vi "VLC-IP_Enqueue_Images.vi"(0 "VLC-IP":T1, 1 "dTime":refnum<vi>, 5 "Stop in":refnum<vi>, 7 "queue in":refnum<queue>, 11 "error in (no error)":errorcluster) -> (15 "error out":errorcluster)   [LabVIEW 2016]
uses:
  <vilib>/vision/Image Controls.llb/IMAQ Image.ctl
  VLC-IP.ctl
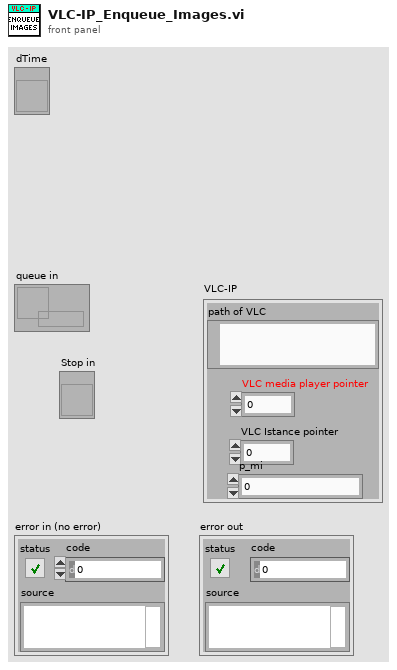
[diagram p1: front panel]
types:
  T1 = typedef "VLC-IP.ctl" = cluster{"path of VLC":path, "VLC media player pointer":i32, "VLC Istance pointer":i32, "p_mi":i32}
  T2 = typedef "Image Type" = u32
  T3 = typedef "IMAQ Image.ctl" = refnum<image>
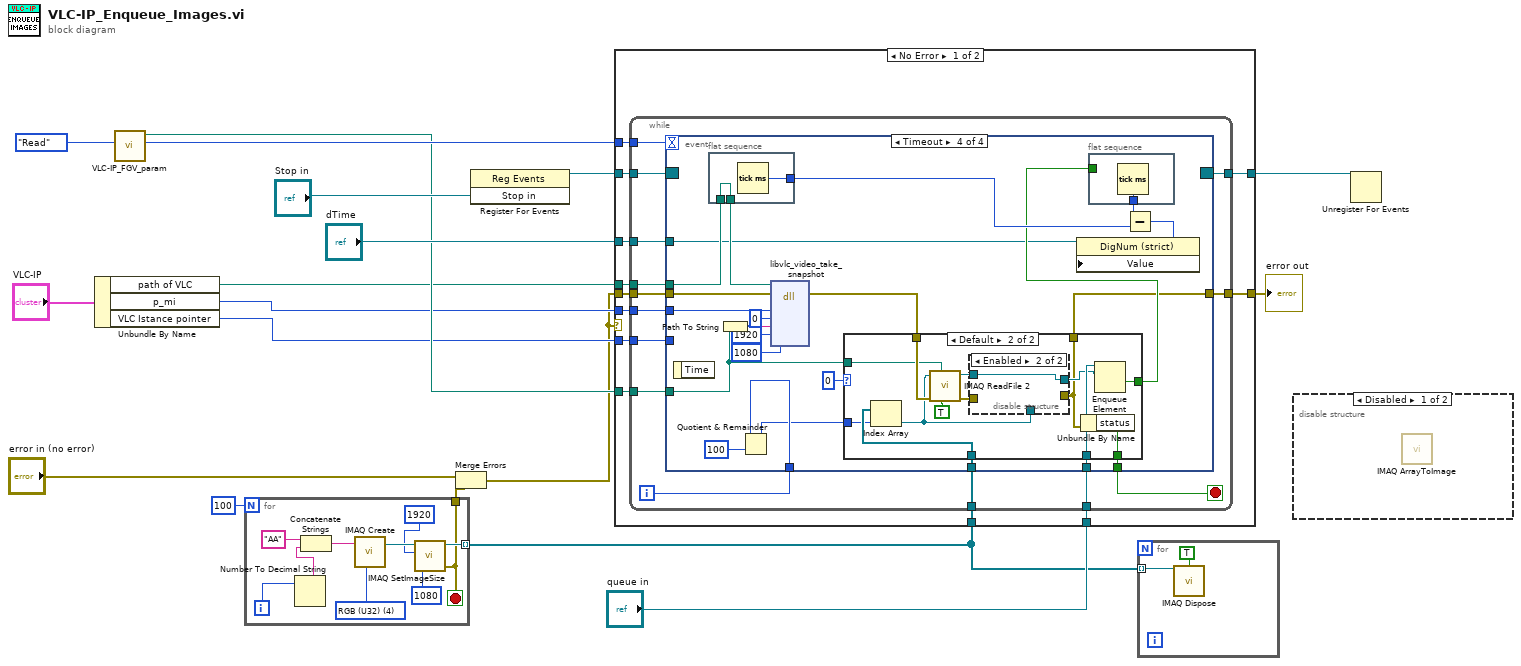
[diagram p0: block diagram]
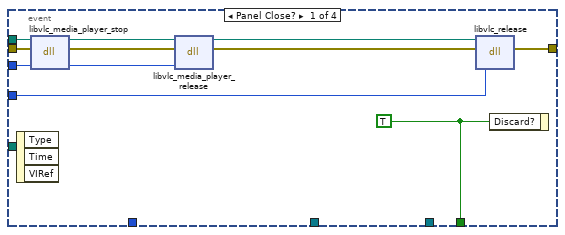
[diagram p3: hidden frame]
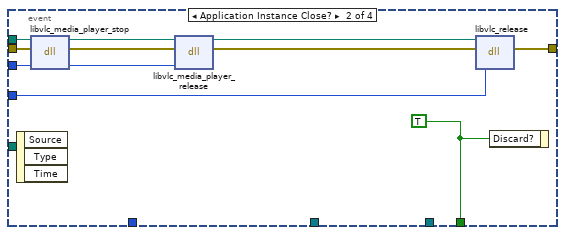
[diagram p4: hidden frame]
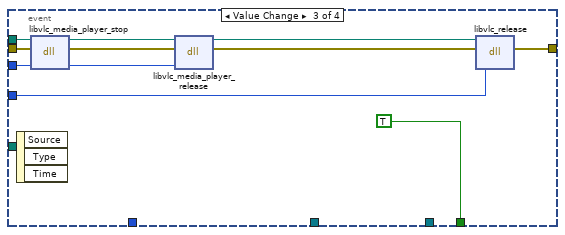
[diagram p5: hidden frame]
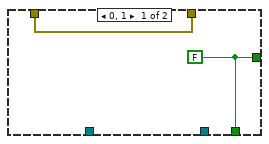
[diagram p6: hidden frame]
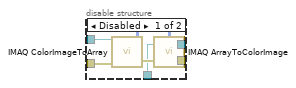
[diagram p7: hidden frame]
diagram:
  n1 = Unbundle By Name("VLC-IP") -> ("path of VLC"=w7:path, "p_mi"=w5:i32, "VLC Istance pointer"=w6:i32)
  n2 = call "VLC-IP_FGV_param.vi"("Mode"=enum16{"Read", "Write"}."Read") -> ("SamplingTime_out"=w10:i32, "TemporaryFilePath_out"=w9:path)  [unwired: 9 in]
  n3 = for {
    N: 100 -> [_]
    tunnel: [w22] -> w3 mode=indexing
    tunnel: [w19] -> w1
    i -> [w24]
    stop <- w19 stop-if-true
    w28 = T2 4 items=["Grayscale (U8)", "Grayscale (I16)", "Grayscale (SGL)", "Complex (CSG)", "RGB (U32)", "HSL (U32)", "RGB (U64)", "Grayscale (U16)"] ("Image Type")
    n4 = Number To Decimal String(number=w24) -> (decimal integer string=w25:string)  [unwired: 1 in]
    n5 = Concatenate Strings("AA" ("Image Name"), w25) -> (w26:string)
    n6 = call "IMAQ Create"("Image Name"=w26, "Image Type"=w28) -> ("New Image"=w21:T3)  [unwired: 3 in, 1 out]
    n7 = call "IMAQ SetImageSize"("Y Resolution"=1080, "X Resolution"=1920, "Image"=w21) -> ("error out"=w19:errorcluster, "Image Out"=w22:T3)  [unwired: 2 in]
  }
  n8 = Merge Errors("error in (no error)", w1) -> (w2:errorcluster)
  n9 = register-events("Stop in") -> (reference out=w15:refnum<event-registration>)  [unwired: 2 in, 1 out]
  n10 = case shown="No Error" w2 {
    tunnel: w6 -> [w40 _]
    tunnel: w5 -> [w39 _]
    tunnel: w2 -> [w38 w138]
    tunnel: w7 -> [w37 _]
    tunnel: [w36 w138] -> w12
    tunnel: w9 -> [w35 _]
    tunnel: w3 -> [w34 _]
    tunnel: "queue in" -> [w33 _]
    tunnel: w10 -> [w32 _]
    tunnel: w15 -> [w31 w137]
    tunnel: [w30 w137] -> w16
    tunnel: "dTime" -> [w29 _]
    frame No Error {
      n11 = while {
        tunnel: w40 -> [w54]
        tunnel: w39 -> [w53]
        tunnel: w38 -> [w52]
        tunnel: w37 -> [w51]
        tunnel: [w50] -> w36
        tunnel: w35 -> [w48]
        tunnel: w34 -> [w47]
        tunnel: w33 -> [w46]
        tunnel: w32 -> [w44]
        tunnel: w31 -> [w43]
        tunnel: [w42] -> w30
        tunnel: w29 -> [w41]
        i -> [w45]
        stop <- w49 stop-if-true
        n12 = event shown="[3] Timeout" {
          selector: w43 -> [_ _ _ _]
          dyn-events: [_ _ _ _] -> w42
          timeout: w44 -> [_ _ _ _]
          tunnel: w52 -> [w65 w76 w87 w106]
          tunnel: w53 -> [w64 w75 w86 w105]
          tunnel: w54 -> [w60 w71 w82 _]
          tunnel: w51 -> [w59 w70 w81 w98]
          tunnel: [w56 w67 w78 w89] -> w50
          tunnel: [w55 w66 TRUE ("Discard?") w90] -> w49
          tunnel: w48 -> [_ _ _ w99]
          tunnel: w47 -> [_ _ _ w101]
          tunnel: w46 -> [_ _ _ w100]
          tunnel: w45 -> [_ _ _ w93]
          tunnel: w41 -> [_ _ _ w95]
          event Panel Close? {
            w55 = TRUE ("Discard?")
            n13 = event-data() -> ()  [unwired: 1 in, 3 out]
            n14 = dll-call lib="C:/Program Files (x86)/VideoLAN/VLC/libvlc.dll" fn="libvlc_media_player_stop"(path in=w59, error in=w65, "p_mi"=w64) -> (path out=w58:path, error out=w63:errorcluster, "p_mi"=w62:i32)  [unwired: 2 in]
            n15 = dll-call lib="C:/Program Files (x86)/VideoLAN/VLC/libvlc.dll" fn="libvlc_media_player_release"(path in=w58, error in=w63, "p_mi"=w62) -> (path out=w57:path, error out=w61:errorcluster)  [unwired: 3 in]
            n16 = dll-call lib="C:/Program Files (x86)/VideoLAN/VLC/libvlc.dll" fn="libvlc_release"(path in=w57, error in=w61, "p_instnace"=w60) -> (error out=w56:errorcluster)  [unwired: 3 in, 1 out]
            n17 = event-data("Discard?"=w55) -> ()  [unwired: 1 in, 1 out]
          }
          event Application Instance Close? {
            w66 = TRUE ("Discard?")
            n18 = event-data() -> ()  [unwired: 1 in, 3 out]
            n19 = dll-call lib="C:/Program Files (x86)/VideoLAN/VLC/libvlc.dll" fn="libvlc_media_player_stop"(path in=w70, error in=w76, "p_mi"=w75) -> (path out=w69:path, error out=w74:errorcluster, "p_mi"=w73:i32)  [unwired: 2 in]
            n20 = dll-call lib="C:/Program Files (x86)/VideoLAN/VLC/libvlc.dll" fn="libvlc_media_player_release"(path in=w69, error in=w74, "p_mi"=w73) -> (path out=w68:path, error out=w72:errorcluster)  [unwired: 3 in]
            n21 = dll-call lib="C:/Program Files (x86)/VideoLAN/VLC/libvlc.dll" fn="libvlc_release"(path in=w68, error in=w72, "p_instnace"=w71) -> (error out=w67:errorcluster)  [unwired: 3 in, 1 out]
            n22 = event-data("Discard?"=w66) -> ()  [unwired: 1 in, 1 out]
          }
          event Value Change {
            n23 = event-data() -> ()  [unwired: 1 in, 3 out]
            n24 = dll-call lib="C:/Program Files (x86)/VideoLAN/VLC/libvlc.dll" fn="libvlc_media_player_stop"(path in=w81, error in=w87, "p_mi"=w86) -> (path out=w80:path, error out=w85:errorcluster, "p_mi"=w84:i32)  [unwired: 2 in]
            n25 = dll-call lib="C:/Program Files (x86)/VideoLAN/VLC/libvlc.dll" fn="libvlc_media_player_release"(path in=w80, error in=w85, "p_mi"=w84) -> (path out=w79:path, error out=w83:errorcluster)  [unwired: 3 in]
            n26 = dll-call lib="C:/Program Files (x86)/VideoLAN/VLC/libvlc.dll" fn="libvlc_release"(path in=w79, error in=w83, "p_instnace"=w82) -> (error out=w78:errorcluster)  [unwired: 3 in, 1 out]
          }
          event Timeout {
            n27 = event-data() -> ()  [unwired: 1 in, 1 out]
            n28 = flat-sequence {
              tunnel: [w135] -> w97
              tunnel: w98 -> [w135]
              tunnel: [w136] -> w103
              frame #0 {
                n29 = Tick Count (ms)() -> (millisecond timer value=w136:u32)
              }
            }
            n30 = Path To String(path=w99) -> (string=w108:string)
            n31 = Quotient & Remainder(x=w93, y=100) -> (x-y*floor(x/y)=w91:i32)  [unwired: 1 out]
            n32 = dll-call lib="C:/Program Files (x86)/VideoLAN/VLC/libvlc.dll" fn="libvlc_video_take_snapshot"(path in=w97, error in=w106, "p_mi"=w105, "num"=u32 0, "psz_filepath"=w108, "i_width"=u32 1920, "i_height"=u32 1080) -> (error out=w102:errorcluster)  [unwired: 7 in, 1 out]
            n33 = case shown="Default" 0 {
              tunnel: w102 -> [w111 w125]
              tunnel: w101 -> [_ w120]
              tunnel: w100 -> [_ w124]
              tunnel: w99 -> [_ w123]
              tunnel: [w112 w122] -> w96
              tunnel: w91 -> [_ w119]
              tunnel: [w112 w114] -> w90
              tunnel: [w111 w113] -> w89
              frame 0, 1 {
                w112 = FALSE ("timed out?")
              }
              frame Default {
                n34 = Index Array(array=w120, index=w119) -> (element=w116:T3)
                n35 = call "IMAQ ReadFile 2"("Use File Path Image Type"=TRUE, "File Path"=w123, "error in (no error)"=w125, "Image"=w116) -> ("error out"=w118:errorcluster, "Image Out"=w117:T3)  [unwired: 3 in, 3 out]
                n36 = disable-structure shown="Enabled" {
                  disable-tunnel: w118 -> [w132 _]
                  disable-tunnel: w117 -> [w131 w133]
                  disable-tunnel: w116 -> [w128 _]
                  disable-tunnel: [w127 w133] -> w115
                  disable-tunnel: [w126 _] -> w113
                  frame Disabled {
                    n37 = call "IMAQ ColorImageToArray"("Image"=w131, "error in (no error)"=w132) -> ("Image Pixels (U32)"=w129:u32[][], "error out"=w130:errorcluster)  [unwired: 2 in, 1 out]
                    n38 = call "IMAQ ArrayToColorImage"("Image Pixels (U32)"=w129, "Image"=w128, "error in (no error)"=w130) -> ("Image Out"=w127:T3, "error out"=w126:errorcluster)  [unwired: 2 in]
                  }
                  frame Enabled {
                  }
                }
                n39 = Unbundle By Name(w113) -> ("status"=w114:bool)
                n40 = Enqueue Element(queue=w124, element=w115) -> (timed out?=w122:bool)  [unwired: 2 in, 2 out]
              }
            }
            n41 = flat-sequence {
              tunnel: w96 -> [_]
              tunnel: [w134] -> w104
              frame #0 {
                n42 = Tick Count (ms)() -> (millisecond timer value=w134:u32)
              }
            }
            n43 = Subtract(x=w104, y=w103) -> (x-y=w94:u32)
            n44 = property class="DigNum (strict)"(reference=w95, "Value"=w94) -> ()  [unwired: 1 in, 2 out]
          }
        }
      }
    }
    frame Error {
    }
  }
  "error out" <- w12
  n45 = for {
    tunnel: w3 -> [w140] mode=indexing
    n46 = call "IMAQ Dispose"("All Images? (No)"=TRUE, "Image"=w140) -> ()  [unwired: 4 in, 1 out]
  }
  n47 = disable-structure shown="Disabled" {
    frame Disabled {
      n48 = call "IMAQ ArrayToImage"() -> ()  [unwired: 10 in, 2 out]
    }
    frame Enabled {
    }
  }
  n49 = Unregister For Events(event registration refnum=w16) -> ()  [unwired: 1 in, 1 out]
